vi "Set message.vi"(10 "WampMessage MsgPack":refnum<class "WampMessage MsgPack.lvclass">, 11 "UnregisteredHandler MsgPack in":refnum<class "UnregisteredHandler MsgPack.lvclass">) -> (3 "UnregisteredHandler MsgPack out":refnum<class "UnregisteredHandler MsgPack.lvclass">)   [LabVIEW 2020, in "wamplv.lvlib" / "UnregisteredHandler MsgPack.lvclass"]
uses:
  UnregisteredHandler MsgPack.lvclass
  UnregisteredHandler MsgPack.lvclass/UnregisteredHandler MsgPack.ctl
  SerialisedMessages/MsgPackMessage/WampMessage MsgPack.lvclass
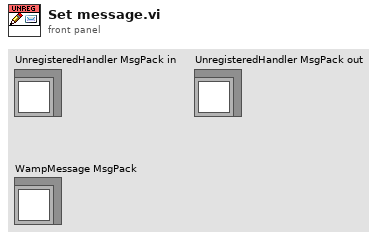
[diagram p1: front panel]
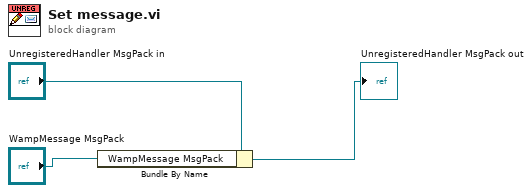
[diagram p0: block diagram]
diagram:
  n1 = Bundle By Name(cluster="UnregisteredHandler MsgPack in", "WampMessage MsgPack"="WampMessage MsgPack") -> (→"UnregisteredHandler MsgPack out":refnum<class "UnregisteredHandler MsgPack.lvclass">)
